vi "formula resolvente 2.vi"() -> ()   [LabVIEW 2018]
uses:
  <vilib>/Analysis/polynomials.llb/Polynomial Roots (DBL).vi
  <vilib>/Analysis/NI_AALPro.lvlib
panel:
  out "Se for imaginário":cdb[](array[numeric])
  in  "Calcular":bool
  out "x2":dbl
  out "x1":dbl
  in  "c":dbl
  in  "b":dbl
  in  "a":dbl
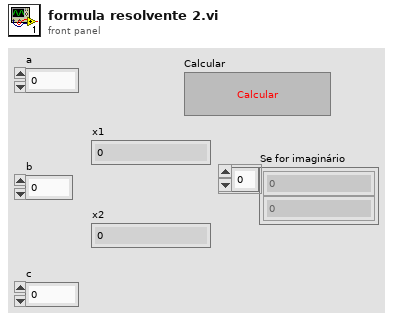
[diagram p1: front panel]
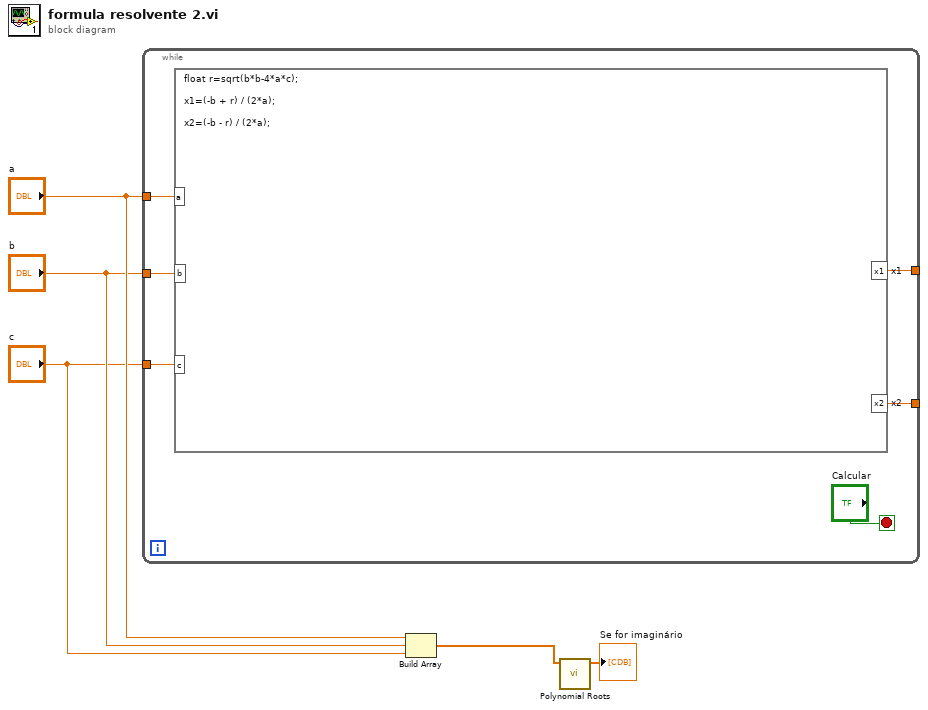
[diagram p0: block diagram]
diagram:
  n1 = while {
    tunnel: "a" -> [w13]
    tunnel: "b" -> [w12]
    tunnel: "c" -> [w11]
    tunnel: [w10] -> w7
    tunnel: [w8] -> w6
    stop <- "Calcular" stop-if-true
    n2 = formula code="float r=sqrt(b*b-4*a*c);\n\nx1=(-b + r) / (2*a);\n\nx2=(-b - r) / (2*a);"("a"=w13, "b"=w12, "c"=w11) -> ("x1"=w8:dbl, "x2"=w10:dbl)
  }
  "x1" <- w6
  "x2" <- w7
  n3 = Build Array("a", "b", "c") -> (w1:dbl[])
  n4 = call-poly <vilib>:"Polynomial Roots.vi"("P(x)"=w1) -> ("Roots"=→"Se for imaginário":cdb[])  [unwired: 9 in, 1 out]
